vi "GFITS_PreviewHeaders.vi"(0 "file":path, 1 "Database RefNum in":T1, 9 "extension":i32=-1, 11 "error in (no error)":errorcluster, 12 "timing":string="after", 13 "nd queue":bool) -> (6 "headers out":string[][](table), 15 "error out":errorcluster)   [LabVIEW 2016]
uses:
  DBSHAND/private/vis/DatabaseHand_RefNum.ctl
  GFITS_Gbls.vi
  DBSHAND/private/vis/DatabaseHand_Element_Get(bool).vi
  DBSHAND/private/vis/DatabaseHand_Element_Get(I32).vi
  DBSHAND/private/vis/DatabaseHand_Element_Get(string).vi
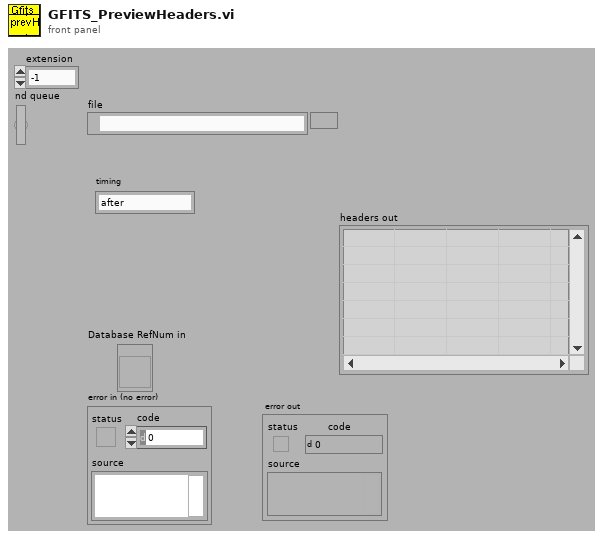
[diagram p1: front panel]
types:
  T1 = typedef "DatabaseHand_RefNum.ctl" = refnum<vi>
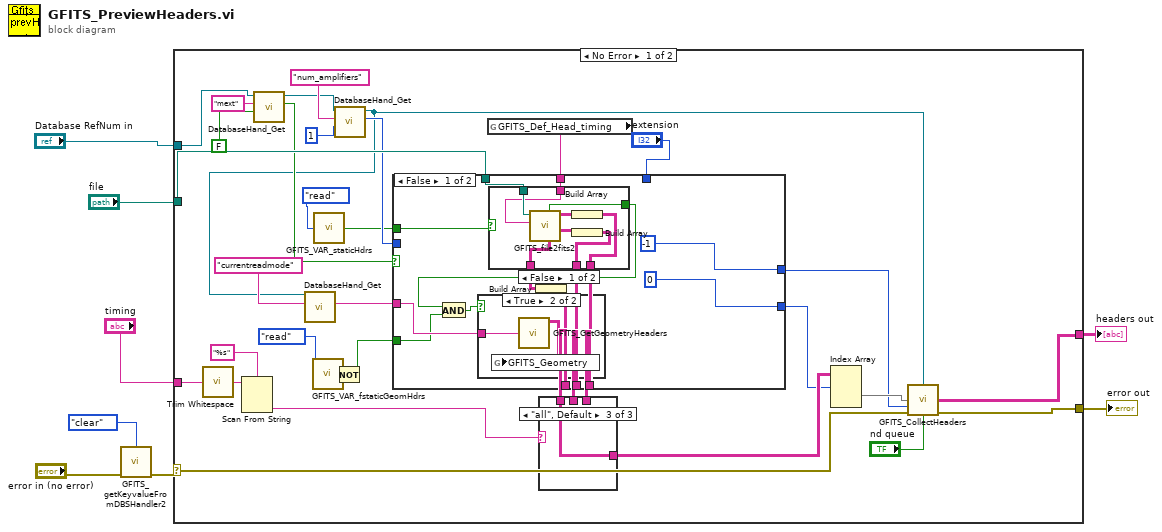
[diagram p0: block diagram]
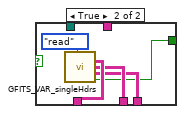
[diagram p3: hidden frame]
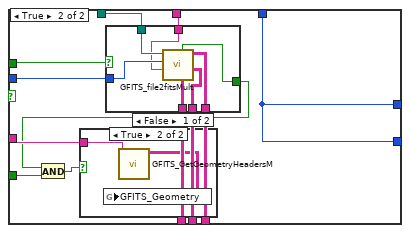
[diagram p4: hidden frame]
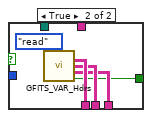
[diagram p6: hidden frame]
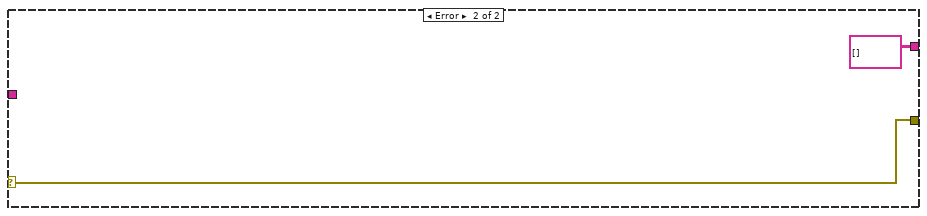
[diagram p9: hidden frame]
diagram:
  n1 = call "GFITS_getKeyvalueFromDBSHandler2.vi"("action"=enum16{"get", "clear"}."clear", "error in (no error)"="error in (no error)") -> ("error out"=w3:errorcluster)  [unwired: 7 in, 6 out]
  n2 = case shown="No Error" w3 {
    selector: w3 -> [w40 w101]
    tunnel: "file" -> [w42 _]
    tunnel: "timing" -> [w18 _]
    tunnel: [w41 w101] -> w5
    tunnel: "Database RefNum in" -> [w29 _]
    tunnel: [w36 string[][] [] ("headers out")] -> w1
    frame No Error {
      n3 = call <vilib>:"Trim Whitespace.vi"("string"=w18) -> ("trimmed string"=w15:string)  [unwired: 1 in]
      n4 = Scan From String(format string="%s", input string=w15) -> (output 1=w16:string)  [unwired: 2 in, 4 out]
      n5 = call-poly "DatabaseHand_Get.vi"("default value"=FALSE, "name"="mext", "Database RefNum in"=w29) -> ("value"=w28:bool, "Database RefNum out"=w31:T1)  [unwired: 2 in, 5 out]
      n6 = call "GFITS_VAR_fstaticGeomHdrs.vi"("action"=enum16{"read", "write"}."read") -> ("static out"=w10:bool)  [unwired: 1 in, 13 out]
      n7 = call "GFITS_VAR_staticHdrs.vi"("action"=enum16{"read", "write"}."read") -> ("static out"=w12:bool)  [unwired: 1 in, 13 out]
      n8 = Not(x=w10) -> (.not. x?=w9:bool)
      n9 = call-poly "DatabaseHand_Get.vi"("default value"=1, "name"="num_amplifiers", "Database RefNum in"=w31) -> ("value"=w27:i32, "Database RefNum out"=w20:T1)  [unwired: 2 in, 5 out]
      n10 = call-poly "DatabaseHand_Get.vi"("name"="currentreadmode", "Database RefNum in"=w20) -> ("value"=w19:string)  [unwired: 3 in, 6 out]
      n11 = global read "GFITS_Gbls.vi" "GFITS_Def_Head_timing"() -> (w35:string)
      n12 = case shown="False" w28 {
        tunnel: w42 -> [w55 w81]
        tunnel: [w50 w77] -> w39
        tunnel: [w53 w79] -> w38
        tunnel: [w52 w78] -> w37
        tunnel: w35 -> [w54 w80]
        tunnel: w27 -> [_ w82]
        tunnel: "extension" -> [_ w76]
        tunnel: [i16 0 ("extension") w76] -> w23
        tunnel: [i16 -1 ("extension") w76] -> w22
        tunnel: w19 -> [w47 w75]
        tunnel: w12 -> [w46 w74]
        tunnel: w9 -> [w43 w71]
        frame False {
          n13 = case shown="False" w46 {
            tunnel: w55 -> [w65 _]
            tunnel: w54 -> [w64 _]
            tunnel: [w63 w67] -> w53
            tunnel: [w60 w68] -> w52
            tunnel: [w59 w69] -> w51
            tunnel: [w58 w66] -> w45
            frame False {
              n14 = call "GFITS_file2fits2.vi"("def_timing"=w64, "file"=w65) -> ("before Keywords"=w61:string[][], "after Keywords"=w62:string[][], "all keys"=w59:string[][], "geominfo?"=w58:bool)  [unwired: 6 out]
              n15 = Build Array(w62) -> (w63:string[][][])
              n16 = Build Array(w61) -> (w60:string[][][])
            }
            frame True {
              n17 = call "GFITS_VAR_singleHdrs.vi"("action"=enum16{"read", "write"}."read") -> ("GFITS_allkeys"=w69:string[][], "GFITS_before"=w68:string[][][], "GFITS_after"=w67:string[][][], "geom info"=w66:bool)  [unwired: 6 in, 5 out]
            }
          }
          n18 = And(x=w45, y=w43) -> (x .and. y?=w44:bool)
          n19 = case shown="True" w44 {
            tunnel: w47 -> [_ w57]
            frame False {
            }
            frame True {
              n20 = call "GFITS_GetGeometryHeaders.vi"("readmode"=w57) -> ("Keywords out"=w56:string[][][])  [unwired: 10 out]
              n21 = global write "GFITS_Gbls.vi" "GFITS_Geometry"(w56) -> ()
            }
          }
          n22 = Build Array(w51) -> (w50:string[][][])
        }
        frame True {
          n23 = case shown="False" w74 {
            tunnel: w82 -> [w91 _]
            tunnel: w81 -> [w90 _]
            tunnel: w80 -> [w89 _]
            tunnel: [w88 w93] -> w79
            tunnel: [w87 w94] -> w78
            tunnel: [w86 w95] -> w77
            tunnel: [w85 w92] -> w73
            frame False {
              n24 = call "GFITS_file2fitsMult.vi"("def_timing"=w89, "number of Extensions"=w91, "filename"=w90) -> ("before keys"=w87:string[][][], "Keywords"=w88:string[][][], "all keys"=w86:string[][][], "geominfo?"=w85:bool)  [unwired: 5 out]
            }
            frame True {
              n25 = call "GFITS_VAR_Hdrs.vi"("action"=enum16{"read", "write"}."read") -> ("GFITS_allkeys"=w95:string[][][], "GFITS_before"=w94:string[][][], "GFITS_after"=w93:string[][][], "geom info"=w92:bool)  [unwired: 6 in, 5 out]
            }
          }
          n26 = And(x=w73, y=w71) -> (x .and. y?=w72:bool)
          n27 = case shown="True" w72 {
            tunnel: w75 -> [_ w84]
            frame False {
            }
            frame True {
              n28 = call "GFITS_GetGeometryHeadersM.vi"("readmode"=w84) -> ("Keywords out"=w83:string[][][])  [unwired: 10 out]
              n29 = global write "GFITS_Gbls.vi" "GFITS_Geometry"(w83) -> ()
            }
          }
        }
      }
      n30 = case shown="\"all\", Default" w16 {
        tunnel: w39 -> [_ _ w99]
        tunnel: [w97 w98 w99] -> w26
        tunnel: w38 -> [w97 _ _]
        tunnel: w37 -> [_ w98 _]
        frame "after" {
        }
        frame "before" {
        }
        frame "all", Default {
        }
      }
      n31 = Index Array(array=w26, index (dim 0)=w23) -> (element=w25:string[][])  [unwired: 2 in]
      n32 = call "GFITS_CollectHeaders.vi"("Database RefNum in"=w20, "Keywords"=w25, "extension"=w22, "error in (no error)"=w40, "nd queue"="nd queue") -> ("headers"=w36:string[][], "error out"=w41:errorcluster)  [unwired: 9 out]
    }
    frame Error {
    }
  }
  "error out" <- w5
  "headers out" <- w1
